vi "Set Parameter.vi"(8 "error in (no error)":errorcluster, 10 "Analyze Parameter":refnum<class "Analyze Parameter Base.lvclass">, 11 "Analyze BaseClass in":refnum<class "Analyze BaseClass.lvclass">) -> (0 "error out":errorcluster, 3 "Analyze BaseClass out":refnum<class "Analyze BaseClass.lvclass">)   [LabVIEW 2020, in "Analyze.lvlib" / "Analyze BaseClass.lvlib" / "Analyze BaseClass.lvclass"]
uses:
  Analyze BaseClass.lvclass
  Analyze Parameter/Analyze Parameter Base/Analyze Parameter Base.lvclass
  Analyze BaseClass.lvclass/Analyze BaseClass.ctl
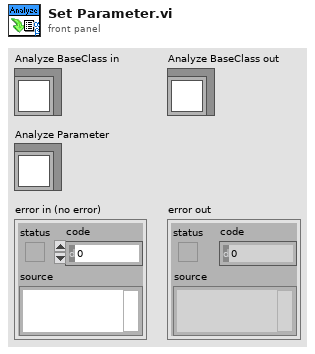
[diagram p1: front panel]
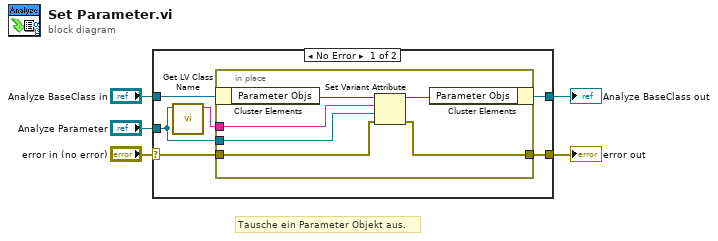
[diagram p0: block diagram]
diagram:
  # "Tausche ein Parameter Objekt aus."
  n1 = case shown="No Error" "error in (no error)" {
    selector: "error in (no error)" -> [w8 w19]
    tunnel: [w7 w19] -> w4
    tunnel: [w6 w18] -> w2
    tunnel: "Analyze BaseClass in" -> [w11 w18]
    tunnel: "Analyze Parameter" -> [w9 _]
    frame No Error {
      n2 = call <vilib>:"Get LV Class Name.vi"("object"=w9) -> ("class name"=w10:string)  [unwired: 9 in, 1 out]
      n3 = in-place {
        in-place-border: w10 -> [w17]
        in-place-border: w9 -> [w16]
        in-place-border: w8 -> [w13]
        in-place-border: [w12] -> w7
        n4 = in-place-cluster #1(w11) -> ("Parameter Objs"=w15:variant)
        n5 = Set Variant Attribute(Variant=w15, name=w17, value=w16, error in=w13) -> (Variant out=w14:variant, error out=w12:errorcluster)  [unwired: 1 out]
        n6 = in-place-cluster #1("Parameter Objs"=w14) -> (w6:refnum<class "Analyze BaseClass.lvclass">)
      }
    }
    frame Error {
    }
  }
  "error out" <- w4
  "Analyze BaseClass out" <- w2
